vi "UMLEditor printWindow.vi"(1 "Picture":picture, 2 "filePath":path, 3 "printToFile":bool) -> ()   [LabVIEW 2016]
doc: "Gets current diagram values"
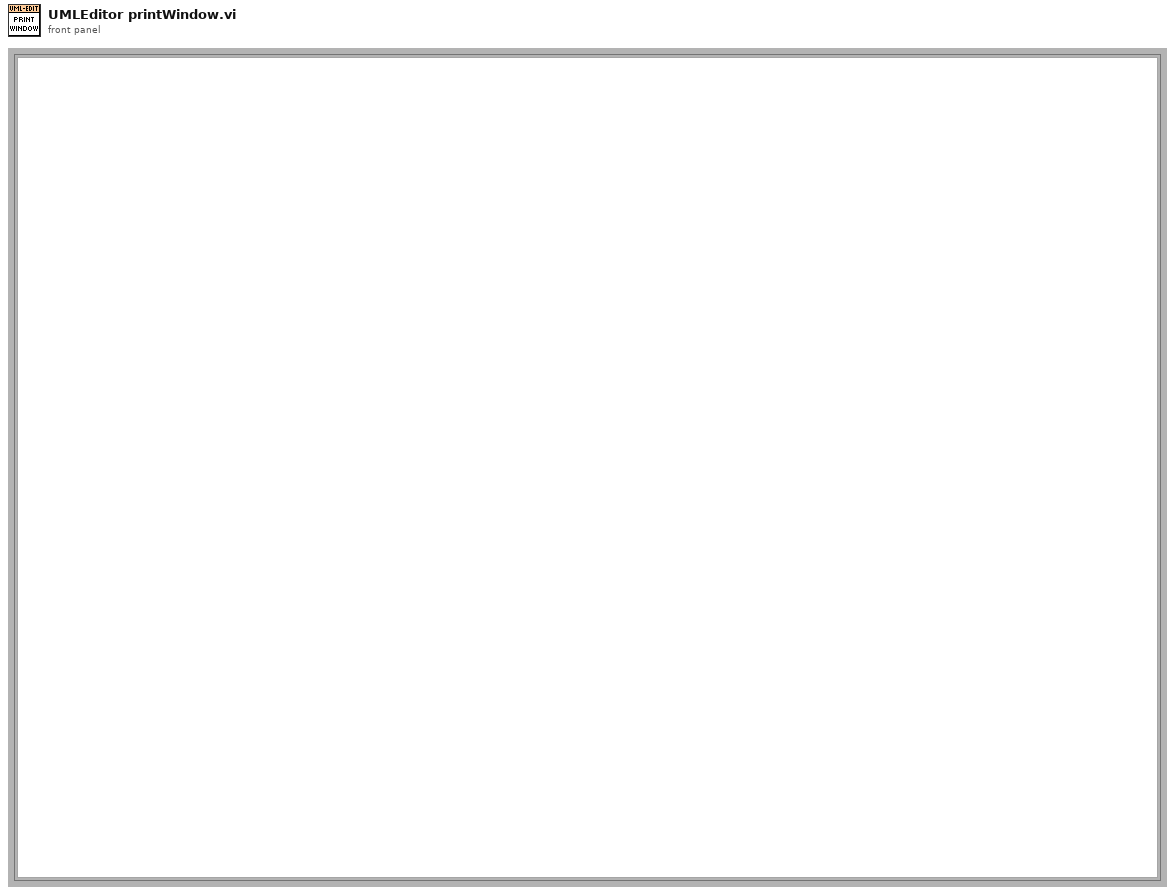
[diagram p1: front panel]
types:
  T1 = typedef "LVBoundsTypeDef.ctl" = cluster{"Width":u32, "Height":u32}
  T2 = typedef "LVRectTypeDef.ctl" = cluster{"left":i16, "top":i16, "right":i16, "bottom":i16}
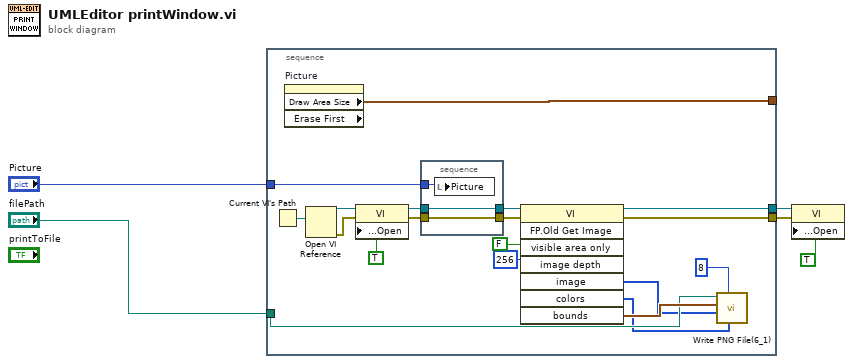
[diagram p0: block diagram]
diagram:
  n1 = stacked-sequence {
    tunnel: "Picture" -> [w20]
    tunnel: [w24] -> _
    tunnel: "filePath" -> [w11]
    tunnel: [w7] -> w3
    tunnel: [w6] -> w2
    frame #0 {
      n2 = Current VI's Path() -> (path=w21:path)
      n3 = property on="Picture" class="Pict" props=["Draw Area Size", "Erase First"]() -> ("Draw Area Size"=w24:T1)  [unwired: 2 in, 3 out]
      n4 = Open VI Reference(vi path=w21) -> (vi reference=w23:refnum<vi>, error out=w22:errorcluster)  [unwired: 1 in, 4 out]
      n5 = property class="VI"(reference=w23, error in=w22, "Front Panel Window:Open"=TRUE) -> (reference out=w19:refnum<vi>, error out=w18:errorcluster)
      n6 = stacked-sequence {
        tunnel: w20 -> [w27]
        tunnel: w19 -> [w26]
        tunnel: w18 -> [w25]
        tunnel: [w26] -> w15
        tunnel: [w25] -> w16
        frame #0 {
          n7 = local write "Picture"(w27) -> ()
        }
      }
      n8 = invoke class="VI" method="FP.Old Get Image"(reference=w15, error in=w16, "visible area only"=FALSE, "image depth"=256) -> (reference out=w7:refnum<vi>, error out=w6:errorcluster, "image"=w10:u8[], "colors"=w9:u32[], "bounds"=w12:T2)  [unwired: 4 in, 3 out]
      n9 = call <vilib>:"Write PNG File(6_1).vi"("color table"=w9, "depth"=u8 8, "flattened image data"=w10, "rect"=w12, "path to PNG file"=w11) -> ()  [unwired: 1 in, 6 out]
    }
  }
  n10 = property class="VI"(reference=w3, error in=w2, "Front Panel Window:Open"=TRUE) -> ()  [unwired: 2 out]
